vi "FF_main_test_devices.vi"() -> ()   [LabVIEW 2016]
uses:
  FF/FF_Read(polymorphic).llb/FF_Read(float).vi
panel:
  in  "xml file":path
  out "Array":sgl[](array[numeric])
  out "x-y":u32
  in  "file path (dialog if empty)":path=path "C:/Documents and Settings/Typhoon 2.5/Desktop/12Xtestbed/Software/data/comm_map.csv"
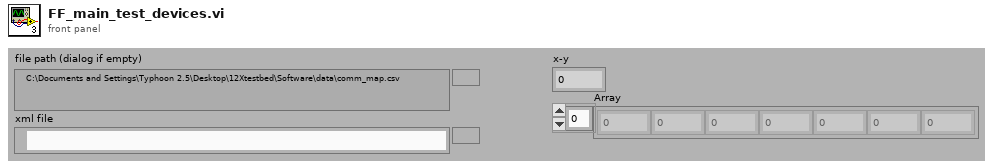
[diagram p1: front panel]
types:
  T1 = typedef "comm_variable_definition.ctl" = cluster{"General Parameter name":string, "MODBUS Register":i32, "Profibus":cluster{"Friendly name":string, "PA":cluster{"Slot":i32, "Index":i32}, "DP":cluster{"Slot":i32, "Index":i32}, "Tag":string}, "Fieldbus":cluster{"Parameter name":string, "Fieldbus Block":string, "Fieldbus Tag":string}, "data type":enum16{"float", "UINT", "UINT32", "STRING"}, "DeviceNET":cluster{"ClassId":u16, "InstanceId":u16, "AttributeId":u8}, "Cluster":T2, "Length":i32}
  T2 = typedef "Comm_mode_and_address_type.ctl" = cluster{"address":i32, "Mode":T3}
  T3 = typedef "Comm_mode_type_combo.ctl" = u16
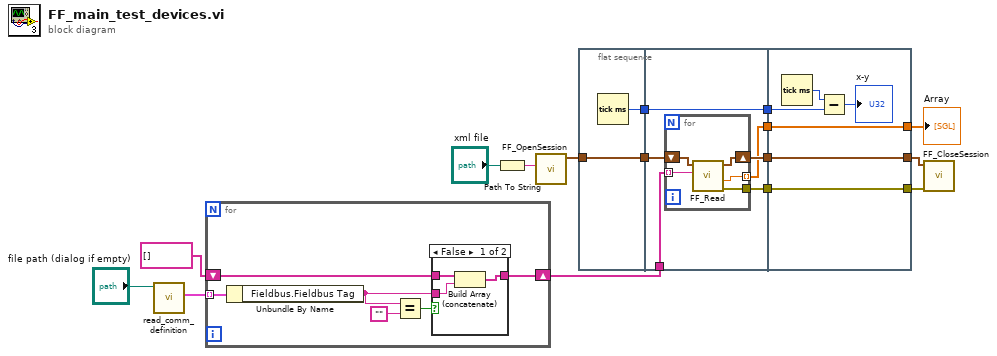
[diagram p0: block diagram]
diagram:
  n1 = call "read_comm_definition.vi"("file path (dialog if empty)"="file path (dialog if empty)") -> ("Comm variable definitions"=w15:T1[])  [unwired: 8 in, 2 out]
  n2 = for {
    tunnel: w15 -> [w22] mode=indexing
    shift-right: [w18] -> w1
    shift-left: string[] [] -> [w17]
    n3 = Unbundle By Name(w22) -> ("Fieldbus.Fieldbus Tag"=w19:string)
    n4 = Equal?(x=w19, y="") -> (x = y?=w20:bool)
    n5 = case shown="False" w20 {
      tunnel: w19 -> [w25 _]
      tunnel: [w24 w26] -> w18
      tunnel: w17 -> [w23 w26]
      frame False {
        n6 = Build Array (concatenate)(w23, w25) -> (w24:string[])
      }
      frame True {
      }
    }
  }
  n7 = Path To String(path="xml file") -> (string=w4:string)
  n8 = call "FF_OpenSession.vi"("tag config file (empty)"=w4) -> ("refnum out"=w2:cluster{"Handle1":u32, "Handle2":u32})  [unwired: 9 in, 1 out]
  n9 = flat-sequence {
    tunnel: w2 -> [w28]
    tunnel: [w28] -> w13
    tunnel: [w27] -> w12
    tunnel: [w34] -> w11
    tunnel: [w33] -> w10
    tunnel: [w32] -> w9
    tunnel: w13 -> [w30]
    tunnel: [w31] -> w8
    tunnel: w12 -> [w31]
    tunnel: w1 -> [w29]
    tunnel: [w43] -> w5
    tunnel: [w44] -> w6
    tunnel: [w45] -> w7
    tunnel: w11 -> [w45]
    tunnel: w10 -> [w44]
    tunnel: w9 -> [w43]
    tunnel: w8 -> [w41]
    frame #0 {
      n10 = Tick Count (ms)() -> (millisecond timer value=w27:u32)
    }
    frame #1 {
      n11 = for {
        tunnel: w29 -> [w39] mode=indexing
        shift-right: [w38] -> w34
        shift-left: w30 -> [w35]
        tunnel: [w37] -> w33
        tunnel: [w36] -> w32 mode=indexing
        n12 = call-poly "FF_Read.vi"("tag"=w39, "refnum in"=w35) -> ("error out"=w37:errorcluster, "value"=w36:sgl, "refnum out"=w38:cluster{"Handle1":u32, "Handle2":u32})  [unwired: 7 in]
      }
    }
    frame #2 {
      n13 = Tick Count (ms)() -> (millisecond timer value=w42:u32)
      n14 = Subtract(x=w42, y=w41) -> (x-y=→"x-y":u32)
    }
  }
  n15 = call "FF_CloseSession.vi"("error in (no error)"=w6, "refnum in"=w7) -> ()  [unwired: 9 in, 1 out]
  "Array" <- w5
